vi "MBThinkDynamicTest.vi"() -> ()   [LabVIEW 2013]
doc: "Use this to get a feel for the MB decision maker in \"real\" time, and test it out, try and find bugs.\n\nFeb. 2014, Eric Schneider"
uses:
  Data/TypeDefs/Boat Regimes.ctl
  Data/TypeDefs/Sailing Regimes.ctl
  Data/TypeDefs/Emergency Regimes.ctl
  Data/TypeDefs/Rudder Set Suggestions.ctl
  Data/TypeDefs/Sail Set Suggestions.ctl
  Utilities/Math/Angles/Angle/Angle.lvclass
panel:
  out "Suggested Sail Setpoints":T1 {"MainSailSuggestion" min=0.0 max=1.0; "JibSailSuggestion" min=0.0 max=1.0}
  out "Suggested Rudder Setpoint":T2 min=-1.0 max=1.0
  out "Heartbeat":bool
  in  "Loop period (ms)":u32(knob)=259 scale=0.0..500.0
  out "Last Commanded Boat Regime":T3={"Sailing Regime"=enum."Upwind - Starboard Tack", "Emergency Regimes"=enum."NO EMERGENCY", "Emergency?"=FALSE}
  in  "Trusted Absolute Wind Data (deg)":dbl(knob)
  in  "Robot Heading (deg)":dbl(knob)
  out "Commanded Boat Regime":T3
  in  "Desired Heading (deg)":dbl(knob)
  in  "stop":bool
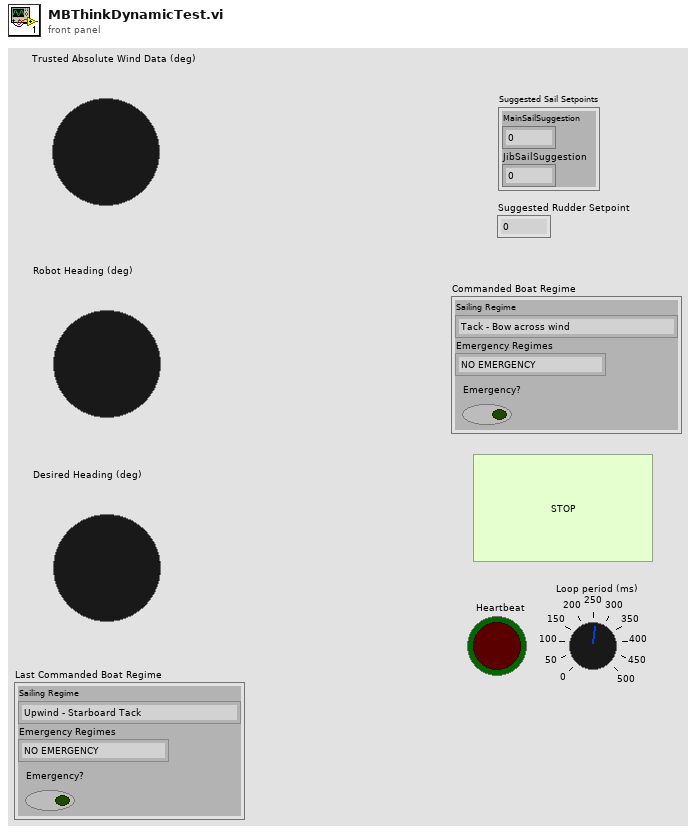
[diagram p1: front panel]
types:
  T1 = typedef "Sail Set Suggestions.ctl" = cluster{"MainSailSuggestion":dbl, "JibSailSuggestion":dbl}
  T2 = typedef "Rudder Set Suggestions.ctl" = dbl
  T3 = typedef "Boat Regimes.ctl" = cluster{"Sailing Regime":T4, "Emergency Regimes":T5, "Emergency?":bool}
  T4 = typedef "Sailing Regimes.ctl" = enum16{"Tack - Bow across wind", "Upwind - Starboard Tack", "Turn between Upwind/Reach - Starboard Tack", "Reach - Starboard Tack", "Turn between Reach/Run - Starboard Tack", "Run - Starboard Tack", "Jibe - Stern across wind", "Run - Port Tack", "Turn between Reach/Run - Port Tack", "Reach - Port Tack", "Turn between Upwind/Reach - Port Tack", "Upwind - Port Tack"}
  T5 = typedef "Emergency Regimes.ctl" = enum16{"NO EMERGENCY", "No Knockdown", "Obstacle Avoid"}
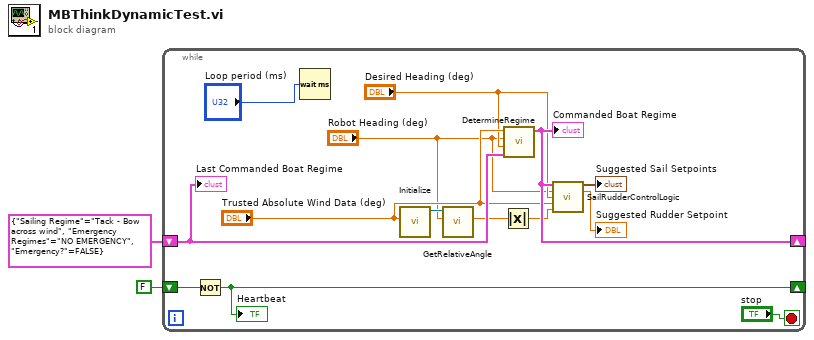
[diagram p0: block diagram]
diagram:
  n1 = while {
    shift-right: [w11] -> _
    shift-left: T3 {"Sailing Regime"=enum."Tack - Bow across wind", "Emergency Regimes"=enum."NO EMERGENCY", "Emergency?"=FALSE} ("Commanded Boat Regime") -> [w15]
    shift-right: [w12] -> _
    shift-left: FALSE -> [w13]
    stop <- "stop" stop-if-true
    n2 = Not(x=w13) -> (.not. x?=w12:bool)
    "Heartbeat" <- w12
    n3 = Wait (ms)(milliseconds to wait="Loop period (ms)") -> ()  [unwired: 1 out]
    n4 = call "Initialize.vi"("Input Angle (Deg.)"="Trusted Absolute Wind Data (deg)") -> ("Angle out"=w9:refnum<class "Angle.lvclass">)  [unwired: 9 in, 1 out]
    n5 = call "GetRelativeAngle.vi"("Boat Heading (Deg.)"="Robot Heading (deg)", "Angle in"=w9) -> ("Relative Angle"=w8:dbl)  [unwired: 8 in, 1 out]
    n6 = Absolute Value(x=w8) -> (abs(x)=w6:dbl)
    n7 = call "DetermineRegime.vi"("Last Commanded Boat Regime"=w15, "Desired Heading (deg)"="Desired Heading (deg)", "Robot Heading (deg)"="Robot Heading (deg)", "Trusted Absolute Wind Data (deg)"="Trusted Absolute Wind Data (deg)") -> ("Commanded Boat Regime"=w11:T3)  [unwired: 7 in]
    "Commanded Boat Regime" <- w11
    n8 = call "SailRudderControlLogic.vi"("Commanded Boat Regime"=w11, "Robot Heading"="Robot Heading (deg)", "DesiredHeading"="Desired Heading (deg)", "AbsoluteWindAngle"="Trusted Absolute Wind Data (deg)", "ApparentWindAngle (0-180)"=w6) -> ("Suggested Sail Setpoints"=→"Suggested Sail Setpoints":T1, "Suggested Rudder Setpoint"=→"Suggested Rudder Setpoint":T2)  [unwired: 9 in]
    "Last Commanded Boat Regime" <- w15
  }
